vi "Main.vi"() -> ()   [LabVIEW 2014, in "Manipulator.lvclass"]
uses:
  Manipulator_class/Manipulator.lvclass
panel:
  in  "CoordinatesIN":cluster{"X":dbl, "Y":dbl, "Z":dbl}
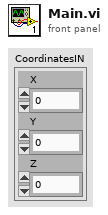
[diagram p1: front panel]
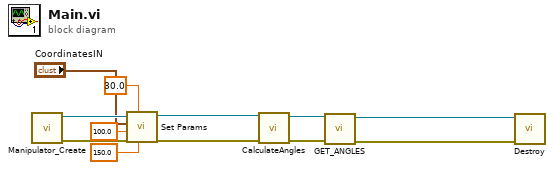
[diagram p0: block diagram]
diagram:
  n1 = call "Manipulator_Create.vi"() -> ("error out"=w11:errorcluster, "reference out"=w12:refnum<class "Manipulator.lvclass">)  [unwired: 10 in]
  n2 = call-dynamic "Set Params.vi"("Lengths.a 2"=150.0, "Lengths.a 3"=30.0, "error in (no error)"=w11, "Lengths.a"=100.0, "CoordinatesIN"="CoordinatesIN", "reference in"=w12) -> ("error out"=w9:errorcluster, "reference out"=w10:refnum<class "Manipulator.lvclass">)  [unwired: 4 in]
  n3 = call "CalculateAngles.vi"("error in (no error)"=w9, "reference in"=w10) -> ("error out"=w8:errorcluster, "reference out"=w5:refnum<class "Manipulator.lvclass">)  [unwired: 8 in]
  n4 = call-dynamic "GET_ANGLES.vi"("error in (no error)"=w8, "reference in"=w5) -> ("error out"=w7:errorcluster, "reference out"=w6:refnum<class "Manipulator.lvclass">)  [unwired: 8 in]
  n5 = call-dynamic "Destroy.vi"("error in (no error)"=w7, "reference in"=w6) -> ()  [unwired: 8 in, 2 out]
